vi "Thermistor.vi"(6 "Units (C)":T1, 7 "Analog Ref Override":dbl, 8 "Error In":errorcluster, 9 "Paired Resistance":i32, 10 "AI Channel":u8, 11 "LINX Resource":T2) -> (0 "Error Out":errorcluster, 2 "Temperature":dbl, 3 "LINX Resource":T2)   [LabVIEW 2019, in "LMH-LINX.lvlib"]
doc: "Read the temperature value from a thermistor."
uses:
  <vilib>/MakerHub/LINX/LMH-LINX.lvlib
  <vilib>/MakerHub/LINX/Private/Type Defs/LINX Ref.ctl
  <vilib>/MakerHub/LINX/Private/Type Defs/Platform.ctl
  <vilib>/MakerHub/LINX/Private/Type Defs/Interface.ctl
  <vilib>/MakerHub/LINX/Private/Device/Type Defs/LINX Device Config.ctl
  <vilib>/MakerHub/LINX/Private/Device/Type Defs/TCP Config.ctl
  <vilib>/MakerHub/LINX/Private/Device/Type Defs/Channels.ctl
  <vilib>/MakerHub/LINX/Private/Type Defs/Temperature Units.ctl
  <vilib>/MakerHub/LINX/Public/Peripherals/Analog/Analog Read 1 Chan.vi
  <vilib>/MakerHub/LINX/Public/Peripherals/Analog/Analog Read N Chans.vi
  <vilib>/MakerHub/LINX/Private/Local IO/LinxAnalogRead.vi
  <vilib>/MakerHub/LINX/Public/Utilities/Check Channel.vi
  <vilib>/MakerHub/LINX/Private/Utilties/Generate Error.vi
  <vilib>/MakerHub/LINX/Private/Device/Device.lvlib
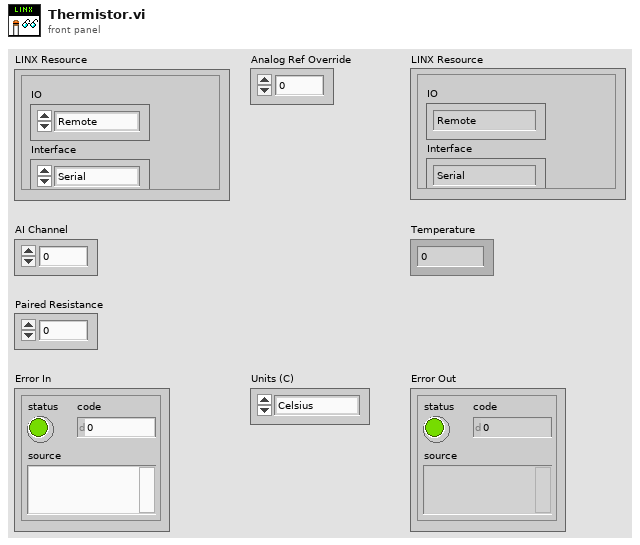
[diagram p1: front panel]
types:
  T1 = typedef "LMH-LINX.lvlib/Temperature Units.ctl" = enum16{"Celsius", "Fahrenheit", "Kelvin", "Rankine"}
  T2 = typedef "LMH-LINX.lvlib/LINX Ref.ctl" = cluster{"IO":T3, "Interface":T4, "LINX Device Config":T5}
  T3 = typedef "LMH-LINX.lvlib/Platform.ctl" = enum16{"Remote", "Local"}
  T4 = typedef "LMH-LINX.lvlib/Interface.ctl" = enum16{"Serial", "TCP"}
  T5 = typedef "LMH-LINX.lvlib/Device.lvlib/LINX Device Config.ctl" = cluster{"Interface":T4, "COM Port":refnum<visa-resource-name>, "TCP Configuration":T6, "Device Family":u8, "Device ID":u8, "Device Name":string, "TCP Ref":refnum<k5>, "Channels":T7}
  T6 = typedef "LMH-LINX.lvlib/Device.lvlib/TCP Config.ctl" = cluster{"IP Address":string, "Port":u16}
  T7 = typedef "LMH-LINX.lvlib/Channels.ctl" = cluster{"DI":u8[], "DO":u8[], "AI":u8[], "AO":u8[], "PWM":u8[], "QE":u8[], "UART":u8[], "I2C 2":u8[], "SPI":u8[], "CAN":u8[], "Servo":u8[], "AI Ref (V)":dbl, "AI Resolution (Bits)":u8, "AO Ref (V)":dbl, "AO Resolution (Bits)":u8}
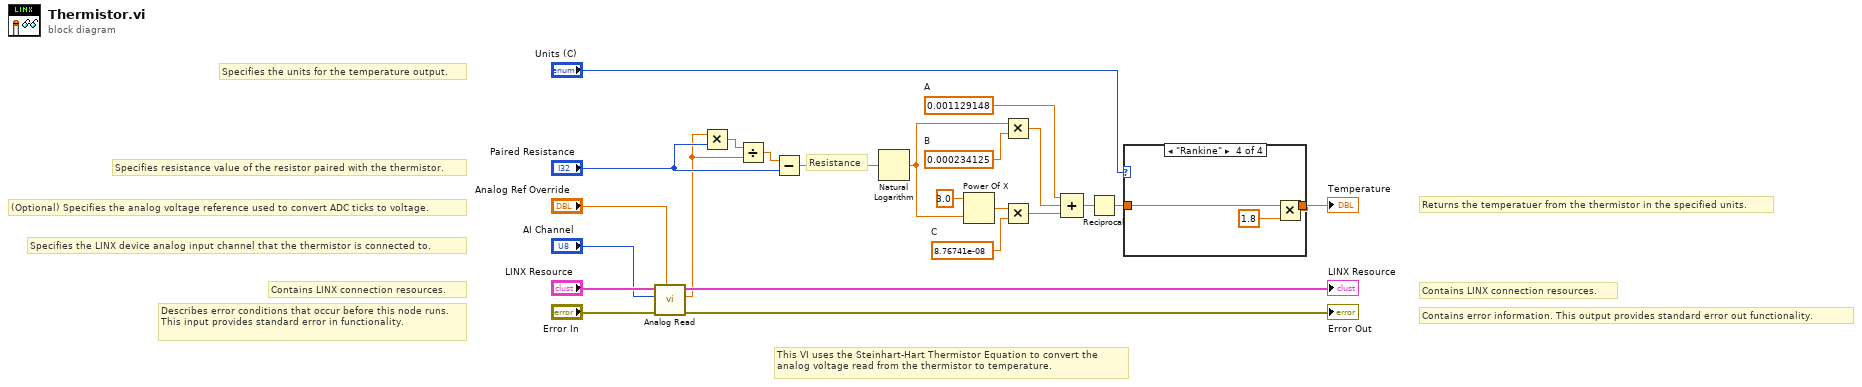
[diagram p0: block diagram]
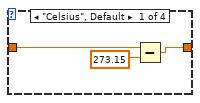
[diagram p2: hidden frame]
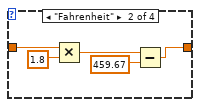
[diagram p3: hidden frame]
diagram:
  w14 = 8.76741e-08  # C
  w11 = 0.001129148  # A
  w16 = 0.000234125  # B
  # "(Optional) Specifies the analog voltage reference used to convert ADC ticks to voltage."
  # "Specifies the LINX device analog input channel that the thermistor is connected to."
  # "Specifies resistance value of the resistor paired with the thermistor."
  # "Specifies the units for the temperature output."
  # "Returns the temperatuer from the thermistor in the specified units."
  # "Contains LINX connection resources."
  # "Contains error information. This output provides standard error out functionality."
  # "Contains LINX connection resources."
  # "Describes error conditions that occur before this node runs. This input provides standard error in functionality."
  # "Resistance"
  # "This VI uses the Steinhart-Hart Thermistor Equation to convert the \nanalog voltage read from the thermistor to temperature."
  n1 = call-poly <vilib>:"Analog Read.vi"("Analog Ref Override (V)"="Analog Ref Override", "Error In"="Error In", "Analog Channel"="AI Channel", "LINX Resource"="LINX Resource") -> ("Error Out"=→"Error Out":errorcluster, "Voltage"=w1:dbl, "LINX Resource"=→"LINX Resource":T2)  [unwired: 4 in, 1 out]
  n2 = Multiply(x=w1, y="Paired Resistance") -> (x*y=w19:dbl)
  n3 = Divide(x=w19, y=w1) -> (x/y=w18:dbl)
  n4 = Subtract(x=w18, y="Paired Resistance") -> (x-y=w17:dbl)
  n5 = Natural Logarithm(1:w17) -> (0:w7:dbl)
  n6 = Power Of X(1:w7, 2:3.0 ("x")) -> (0:w15:dbl)
  n7 = Multiply(x=w7, y=w16) -> (x*y=w12:dbl)
  n8 = Multiply(x=w15, y=w14) -> (x*y=w13:dbl)
  n9 = Compound Arithmetic op=ADD(w11, w12, w13) -> (w10:dbl)
  n10 = Reciprocal(x=w10) -> (1/x=w9:dbl)
  n11 = case shown="\"Rankine\"" "Units (C)" {
    tunnel: w9 -> [w26 w31 w32 w33]
    tunnel: [w24 w27 w32 w35] -> w6
    frame "Celsius", Default {
      n12 = Subtract(x=w26, y=273.15) -> (x-y=w24:dbl)
    }
    frame "Fahrenheit" {
      n13 = Multiply(x=w31, y=1.8) -> (x*y=w29:dbl)
      n14 = Subtract(x=w29, y=459.67) -> (x-y=w27:dbl)
    }
    frame "Kelvin" {
    }
    frame "Rankine" {
      n15 = Multiply(x=w33, y=1.8 ("x")) -> (x*y=w35:dbl)
    }
  }
  "Temperature" <- w6
